vi "dosteps.vi"(8 "error in (no error)":errorcluster, 11 "MSCU":refnum<class "MSCU.lvclass">) -> (0 "error out":errorcluster, 2 "Do Steps":string, 3 "MSCU":refnum<class "MSCU.lvclass">)   [LabVIEW 2019, in "MSCU.lvclass"]
uses:
  MSCU.lvclass
  MSCU.lvclass/MSCU.ctl
panel:
  in  "Steps":i32 min=-1 max=32767 step=1
  in  "Direction":i32 min=-1 max=1 step=2
  in  "Channel":i32=1 min=1 max=8 step=1
  # "1 to 32767 (steps)\n-1 to perform steps continuously\n0 to stop moving"
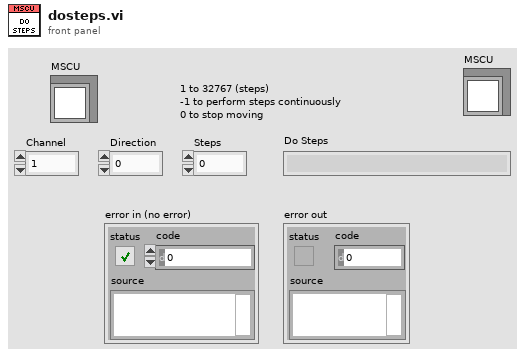
[diagram p1: front panel]
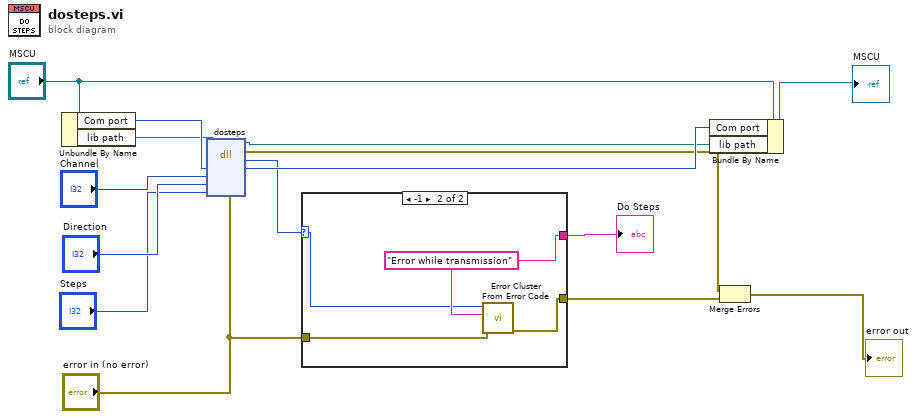
[diagram p0: block diagram]
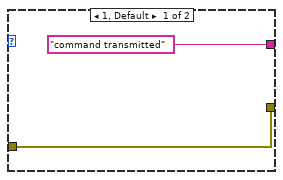
[diagram p2: hidden frame]
diagram:
  n1 = Unbundle By Name("MSCU") -> ("Com port"=w12:i32, "lib path"=w11:path)
  n2 = dll-call lib="C:/Program Files (x86)/Nanonis/SPM Controller/data/MSCU.dll" fn="dosteps"(path in=w11, error in="error in (no error)", "Comport"=w12, "Channel"="Channel", "Direction"="Direction", "Steps"="Steps") -> (path out=w9:path, error out=w5:errorcluster, "return type"=w13:i32, "Comport"=w15:i32)  [unwired: 4 in]
  n3 = case shown="-1" w13 {
    selector: w13 -> [_ w18]
    tunnel: ["command transmitted" w19] -> w14
    tunnel: [w16 w20] -> w3
    tunnel: "error in (no error)" -> [w16 w21]
    frame 1, Default {
    }
    frame -1 {
      w19 = "Error while transmission"
      n4 = call <vilib>:"Error Cluster From Error Code.vi"("error in (no error)"=w21, "error message (\"\")"=w19, "error code (0)"=w18) -> ("error out"=w20:errorcluster)  [unwired: 6 in]
    }
  }
  "Do Steps" <- w14
  n5 = Bundle By Name(cluster="MSCU", "Com port"=w15, "lib path"=w9) -> (→"MSCU":refnum<class "MSCU.lvclass">)
  n6 = Merge Errors(w5, w3) -> (→"error out":errorcluster)
